vi "Drive Off Line.vi"(10 "Start?":bool) -> ()   [LabVIEW 2019]
uses:
  <vilib>/Rock Robotics/WPI/Utilities/WPI_GetSetVariantRefNum.vi
  <vilib>/Rock Robotics/WPI/ThirdParty/Phoenix-LabVIEW/Motor Controller/Sensor/CTRE_Phoenix_MotorControl_SetIntegratedSensorPosition_TalonFX.vi
  <vilib>/Rock Robotics/WPI/RobotDrive/WPI_RobotDriveMecanumDrive_Cartesian.vi
  <vilib>/Rock Robotics/WPI/ThirdParty/Phoenix-LabVIEW/Motor Controller/Get/CTRE_Phoenix_MotorController_GetSelectedSensorData.vi
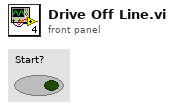
[diagram p1: front panel]
types:
  T1 = typedef "WPI_MotorControlDeviceRef.ctl" = cluster{"DeviceStatus":errorcluster, "Type":T2, "PWM":cluster{"PWM Channel":T3, "DeadBand":T4}, "CAN":cluster{"Device Number":u8, "SetOutput VI Ref":variant, "GetOutput VI Ref":variant, "Enable VI Ref":variant, "Disable VI Ref":variant, "Data":variant}, "Invert":bool, "DIO PWM":cluster{"PWM \"Enable\" Channel":T3, "DIOChannel":T5, "PWM Rate":dbl}}
  T2 = typedef "WPI_MotorControlType.ctl" = enum16{"PWM", "CAN", "DIO PWM"}
  T3 = typedef "FPGA_DIOPWMChannel.ctl" = enum8{"PWM 0", "PWM 1", "PWM 2", "PWM 3", "PWM 4", "PWM 5", "PWM 6", "PWM 7", "PWM 8", "PWM 9", "PWM MXP 0", "PWM MXP 1", "PWM MXP 2", "PWM MXP 3", "PWM MXP 4", "PWM MXP 5", "PWM MXP 6", "PWM MXP 7", "PWM MXP 8", "PWM MXP 9", "Invalid"}
  T4 = typedef "WPI_PWMDeadband.ctl" = cluster{"Name":string, "maxPositivePwm":i32, "minPositivePwm":i32, "centerPwm":i32, "maxNegativePwm":i32, "minNegativePwm":i32, "angularRange":u16}
  T5 = typedef "FPGA_DIOChannel.ctl" = enum8{"DIO 0", "DIO 1", "DIO 2", "DIO 3", "DIO 4", "DIO 5", "DIO 6", "DIO 7", "DIO 8", "DIO 9", "DIO MXP 0", "DIO MXP 1", "DIO MXP 2", "DIO MXP 3", "DIO MXP 4", "DIO MXP 5", "DIO MXP 6", "DIO MXP 7", "DIO MXP 8", "DIO MXP 9", "DIO MXP 10", "DIO MXP 11", "DIO MXP 12", "DIO MXP 13", "DIO MXP 14", "DIO MXP 15", "SPI Port CS1", "SPI Port CS2", "SPI Port CS3", "SPI Port MISO", "SPI Port MOSI", "Invalid"}
  T6 = typedef "WPI_RobotDriveDevRef.ctl" = cluster{"DevStatus":errorcluster, "Motors[]":T1[], "Square Inputs":bool, "Max Output":dbl}
  T7 = typedef "WPI_GyroDevRef.ctl" = cluster{"DevStatus":errorcluster, "Analog Channel":T8, "Gain (VoltsPerDegree/Second)":dbl, "Gyro Type":enum16{"Analog", "XRS450"}, "Handle":i32, "SPI Bus":T9, "Device Found":bool, "Sample Rate":dbl, "Calibrate On Open":bool, "Offset":dbl}
  T8 = typedef "FPGA_AIChannel.ctl" = enum8{"AI 0", "AI 1", "AI 2", "AI 3", "AI MXP 0", "AI MXP 1", "AI MXP 2", "AI MXP 3", "Invalid"}
  T9 = typedef "spi_bus.ctl" = enum16{"SPI On-Board, CS0", "SPI On-Board, CS1", "SPI On-Board, CS2", "SPI On-Board, CS3", "SPI MXP", "Invalid"}
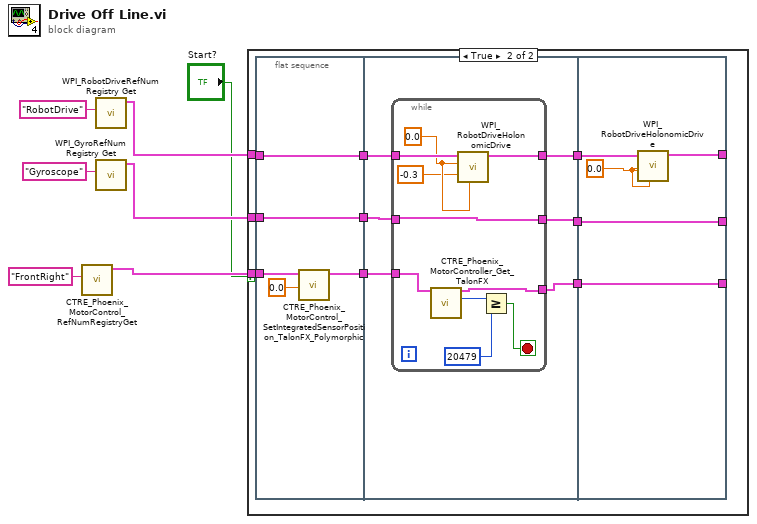
[diagram p0: block diagram]
diagram:
  n1 = call <vilib>:"CTRE_Phoenix_MotorControl_RefNumRegistryGet.vi"("refnum name"="FrontRight") -> ("PhoenixMotorControlDevRef"=w2:T1)  [unwired: 9 in, 1 out]
  n2 = call <vilib>:"WPI_RobotDriveRefNum Registry Get.vi"("refnum name"="RobotDrive") -> ("RobotDriveDevRef"=w4:T6)  [unwired: 9 in, 1 out]
  n3 = call <vilib>:"WPI_GyroRefNum Registry Get.vi"("refnum name"="Gyroscope") -> ("GyroDevRef"=w3:T7)  [unwired: 9 in, 1 out]
  n4 = case shown="True" "Start?" {
    tunnel: w4 -> [_ w10]
    tunnel: w3 -> [_ w9]
    tunnel: w2 -> [_ w8]
    frame False {
    }
    frame True {
      n5 = flat-sequence {
        tunnel: w8 -> [w18]
        tunnel: w9 -> [w20]
        tunnel: w10 -> [w21]
        tunnel: [w21] -> w16
        tunnel: [w20] -> w15
        tunnel: [w19] -> w14
        tunnel: w16 -> [w24]
        tunnel: w15 -> [w25]
        tunnel: w14 -> [w27]
        tunnel: [w26] -> w13
        tunnel: [w23] -> w12
        tunnel: [w22] -> w11
        tunnel: [w42] -> _
        tunnel: w13 -> [w42]
        tunnel: w12 -> [w40]
        tunnel: [w41] -> _
        tunnel: w11 -> [w41]
        tunnel: [w39] -> _
        frame #0 {
          n6 = call-poly <vilib>:"CTRE_Phoenix_MotorControl_SetIntegratedSensorPosition_TalonFX_Polymorphic.vi"("New Position"=0.0, "PhoenixMotorControlDevRef"=w18) -> ("PhoenixMotorControlDevRef"=w19:T1)  [unwired: 8 in, 1 out]
        }
        frame #1 {
          n7 = while {
            tunnel: w27 -> [w35]
            tunnel: [w28] -> w26
            tunnel: w25 -> [w28]
            tunnel: w24 -> [w37]
            tunnel: [w36] -> w23
            tunnel: [w31] -> w22
            stop <- w34 stop-if-true
            w30 = 0.0 ("X")
            n8 = call-poly <vilib>:"CTRE_Phoenix_MotorController_Get_TalonFX.vi"("PhoenixMotorControlDevRef"=w35) -> ("PhoenixMotorControlDevRef"=w31:T1, "Position (Raw Sensor Units)"=w33:i32)  [unwired: 11 in, 2 out]
            n9 = call-poly <vilib>:"WPI_RobotDriveHolonomicDrive.vi"("Rotation"=w30, "Y"=-0.3, "X"=w30, "RobotDriveDevRef"=w37) -> ("RobotDriveDevRef"=w36:T6)  [unwired: 5 in, 2 out]
            n10 = Greater Or Equal?(x=w33, y=20479) -> (x >= y?=w34:bool)
          }
        }
        frame #2 {
          w38 = 0.0 ("X")
          n11 = call-poly <vilib>:"WPI_RobotDriveHolonomicDrive.vi"("Rotation"=w38, "Y"=w38, "X"=w38, "RobotDriveDevRef"=w40) -> ("RobotDriveDevRef"=w39:T6)  [unwired: 5 in, 2 out]
        }
      }
    }
  }
